vi "Write WiringRules[].vi"(10 "WiringRules[]":T1(array[ring]), 11 "PolymorphicInstance in":refnum<class "PolymorphicInstance.lvclass">) -> (3 "PolymorphicInstance out":refnum<class "PolymorphicInstance.lvclass">)   [LabVIEW 2012, in "PolymorphicInstance.lvclass"]
uses:
  PolymorphicInstance.lvclass
  PolymorphicInstance.lvclass/PolymorphicInstance.ctl
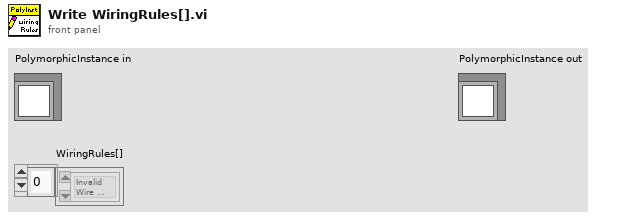
[diagram p1: front panel]
types:
  T1 = enum16{"Invalid Wire Rule", "Required", "Recommended", "Optional", "Dynamic Dispatch"}[]
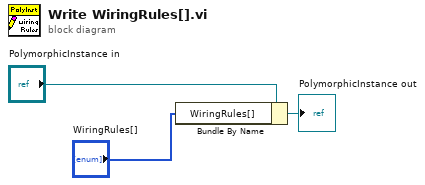
[diagram p0: block diagram]
diagram:
  n1 = Bundle By Name(cluster="PolymorphicInstance in", "WiringRules[]"="WiringRules[]") -> (→"PolymorphicInstance out":refnum<class "PolymorphicInstance.lvclass">)
